vi "Create Antinodes Harmonics.vi"(7 "Max Grid Index":T1, 10 "Antena 2":T1, 11 "Antena 1":T1) -> (3 "Antinodes":T1[](array[typedef]))   [LabVIEW 2024]
uses:
  Cluster_Position.ctl
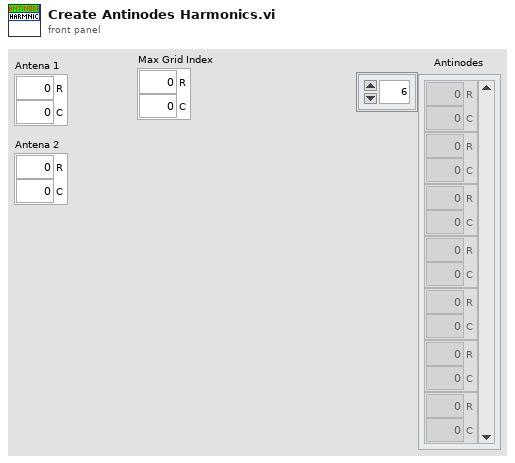
[diagram p1: front panel]
types:
  T1 = typedef "Cluster_Position.ctl" = cluster{"R":i32, "C":i32}
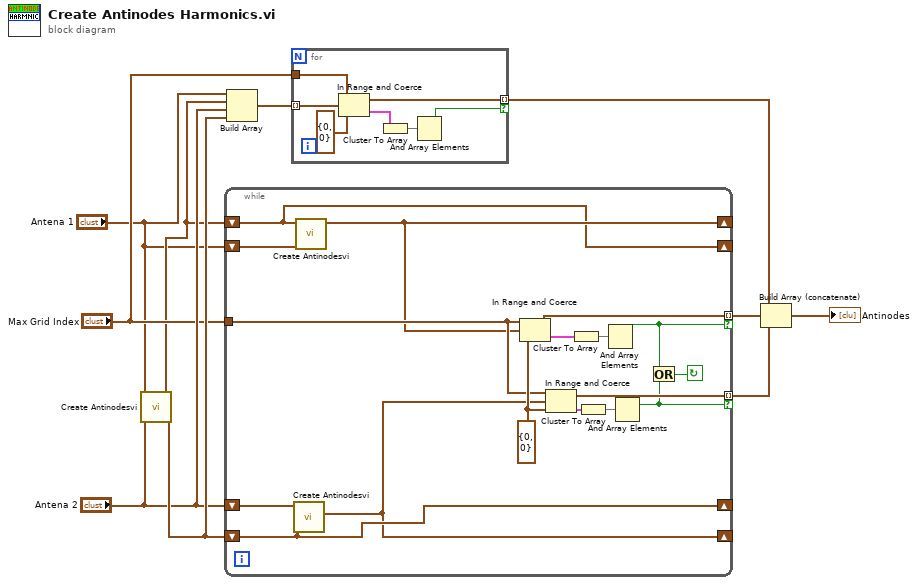
[diagram p0: block diagram]
diagram:
  n1 = call "Create Antinodesvi.vi"("Antena 2"="Antena 2", "Antena 1"="Antena 1") -> ("AntiNode 2 Out"=w7:T1, "AntiNoed 1 Out"=w2:T1)  [unwired: 8 in]
  n2 = while {
    shift-right: [w12] -> _
    shift-left: w2 -> [w11]
    shift-right: [w13] -> _
    shift-left: w7 -> [w14]
    tunnel: [w25] -> w10 mode=indexing if=w18
    tunnel: "Max Grid Index" -> [w23]
    tunnel: [w22] -> w9 mode=indexing if=w19
    shift-right: [w14] -> _
    shift-left: "Antena 2" -> [w16]
    shift-right: [w11] -> _
    shift-left: "Antena 1" -> [w15]
    stop <- w17 continue-if-true
    w24 = T1 {"R"=0, "C"=0}
    n3 = call "Create Antinodesvi.vi"("Antena 2"=w14, "Antena 1"=w16) -> ("AntiNode 2 Out"=w13:T1)  [unwired: 8 in, 1 out]
    n4 = call "Create Antinodesvi.vi"("Antena 2"=w15, "Antena 1"=w11) -> ("AntiNoed 1 Out"=w12:T1)  [unwired: 8 in, 1 out]
    n5 = In Range and Coerce(upper limit=w23, x=w12, lower limit=w24) -> (coerced(x)=w25:T1, In Range?=w26:cluster{"R":bool, "C":bool})
    n6 = In Range and Coerce(upper limit=w23, x=w13, lower limit=w24) -> (coerced(x)=w22:T1, In Range?=w21:cluster{"R":bool, "C":bool})
    n7 = Cluster To Array(cluster=w26) -> (array=w27:bool[])
    n8 = Cluster To Array(cluster=w21) -> (array=w20:bool[])
    n9 = And Array Elements(Boolean array=w27) -> (logical AND=w18:bool)
    n10 = And Array Elements(Boolean array=w20) -> (logical AND=w19:bool)
    n11 = Or(x=w18, y=w19) -> (x .or. y?=w17:bool)
  }
  n12 = Build Array("Antena 1", w2, "Antena 2", w7) -> (w5:T1[])
  n13 = for {
    tunnel: w5 -> [w34] mode=indexing
    tunnel: "Max Grid Index" -> [w33]
    tunnel: [w29] -> w3 mode=indexing if=w28
    n14 = In Range and Coerce(upper limit=w33, x=w34, lower limit=T1 {"R"=0, "C"=0}) -> (coerced(x)=w29:T1, In Range?=w30:cluster{"R":bool, "C":bool})
    n15 = Cluster To Array(cluster=w30) -> (array=w31:bool[])
    n16 = And Array Elements(Boolean array=w31) -> (logical AND=w28:bool)
  }
  n17 = Build Array (concatenate)(w3, w10, w9) -> (→"Antinodes":T1[])
